vi "TEST.vi"() -> ()   [LabVIEW 2013, in "CConfig Object.lvclass"]
doc: "Copyright 2018, Carya Automatisering, Wiebe Walstra."
uses:
  CConfig Object.lvclass
  Delete Query/Delete Query.lvclass
  Data.ctl
  Loop Query/Loop Query.lvclass
  Insert Query/Insert Query.lvclass
  Composite Query/Composite Query.lvclass
  Step In Query/Step In Query.lvclass
  Add Results Query/Add Results Query.lvclass
  Loop Query/Match Query/Match Query.lvclass
panel:
  out "Index 2":i32
  out "Results":string[][](array[string])
  out "error out":errorcluster
  out "String 3":string
  out "String 2":string
  out "Index out":i32
  out "String":string
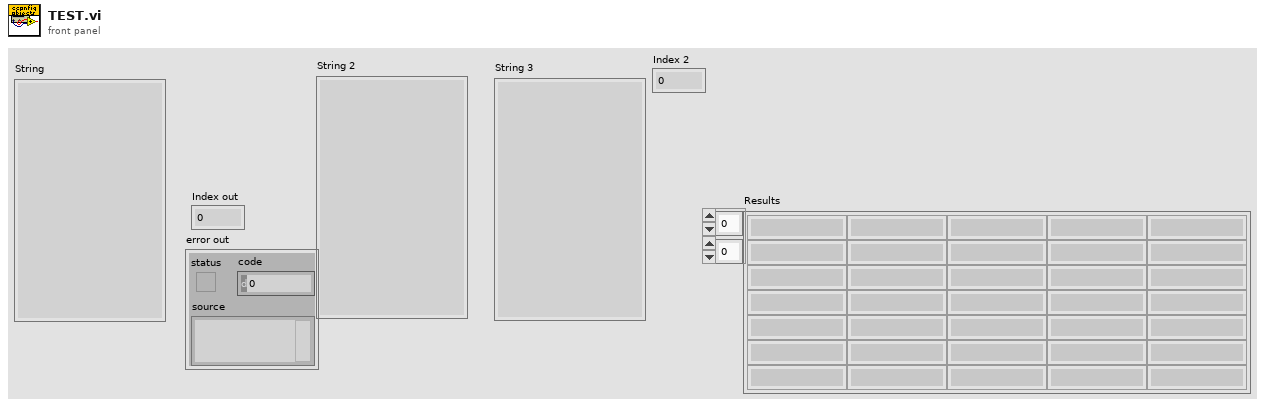
[diagram p1: front panel]
types:
  T1 = typedef "CConfig Object.lvclass/Data.ctl" = enum16{"pre", "name", "middle", "value", "post", "newline", "persistant", "tagged", "type"}
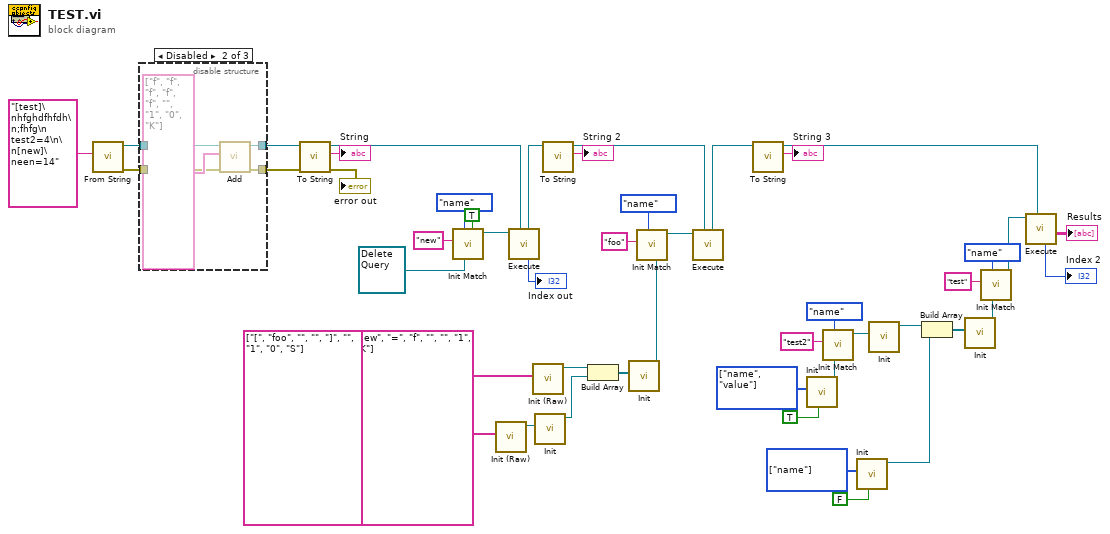
[diagram p0: block diagram]
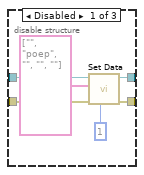
[diagram p2: hidden frame]
diagram:
  w14 = T1[] [enum."name"] items=["pre", "name", "middle", "value", "post", "newline", "persistant", "tagged", "type"] ("Data")
  w26 = T1[] [enum."name", enum."value"] items=["pre", "name", "middle", "value", "post", "newline", "persistant", "tagged", "type"] ("Data")
  n1 = call "From String.vi"("String"="[test]\nhfghdfhfdh\n;fhfg\n test2=4\n\n[new]\neen=14") -> ("error out"=w28:errorcluster, "Section Object out"=w45:refnum<class "CConfig Object.lvclass">)  [unwired: 8 in, 1 out]
  n2 = disable-structure shown="Disabled" {
    disable-tunnel: w45 -> [w53 w58 w60]
    disable-tunnel: [w52 w57 w60] -> w27
    disable-tunnel: [w48 w55 w59] -> w29
    disable-tunnel: w28 -> [w49 w54 w59]
    frame Disabled {
      n3 = call-dynamic "Set Data.vi"("Index in"=1, "error in (no error)"=w49, "Data"=string[] ["", "poep", "", "", ""], "Composite Object in"=w53) -> ("error out"=w48:errorcluster, "Composite Object out"=w52:refnum<class "Config Objects.lvclass">)  [unwired: 6 in]
    }
    frame Disabled {
      n4 = call-dynamic "Add.vi"("error in (no error)"=w54, 10:string[] ["f", "f", "f", "f", "f", "", "1", "0", "K"] ("Data"), "Composite Object in"=w58) -> ("error out"=w55:errorcluster, "Composite Object out"=w57:refnum<class "CConfig Object.lvclass">)  [unwired: 6 in, 1 out]
    }
    frame Enabled {
    }
  }
  n5 = call-dynamic "To String.vi"("error in (no error)"=w29, "Section Object in"=w27) -> ("error out"=→"error out":errorcluster, "String"=→"String":string, "Section Object out"=w1:refnum<class "CConfig Object.lvclass">)  [unwired: 6 in, 1 out]
  n6 = call "Init Match.vi"("Regex [F]"=TRUE, "Found"=refnum<class "Delete Query.lvclass"> refnum ("Delete Query.lvclass"), "Data [name]"=Data."name", "Data"="new") -> ("Find First Query out"=w5:refnum<class "Loop Query.lvclass">)  [unwired: 6 in, 1 out]
  n7 = call "Init (Raw).vi"("Data"=string[] ["", "new", "=", "f", "", "", "1", "0", "K"]) -> ("Find First Query out"=w18:refnum<class "Insert Query.lvclass">)  [unwired: 9 in, 1 out]
  n8 = call-dynamic "Execute.vi"("Composite Object"=w1, "Config Query in"=w5) -> ("Index"=→"Index out":i32, "Composite Object"=w41:refnum<class "CConfig Object.lvclass">)  [unwired: 4 in, 4 out]
  n9 = call "Init (Raw).vi"("Data"=string[] ["[", "foo", "", "", "]", "", "1", "0", "S"]) -> ("Find First Query out"=w32:refnum<class "Insert Query.lvclass">)  [unwired: 9 in, 1 out]
  n10 = call "Init.vi"("Config Query"=w18) -> ("Step In Query out"=w19:refnum<class "Step In Query.lvclass">)  [unwired: 9 in, 1 out]
  n11 = call-dynamic "To String.vi"("Section Object in"=w41) -> ("String"=→"String 2":string, "Section Object out"=w20:refnum<class "CConfig Object.lvclass">)  [unwired: 7 in, 2 out]
  n12 = Build Array(w32, w19) -> (w33:refnum<class "CConfig Query.lvclass">[])
  n13 = call "Init.vi"("Queries"=w33) -> ("Step In Query out"=w34:refnum<class "CConfig Query.lvclass">)  [unwired: 9 in, 1 out]
  n14 = call "Init Match.vi"("Not found"=w34, "Data [name]"=Data."name", "Data"="foo") -> ("Find First Query out"=w4:refnum<class "Loop Query.lvclass">)  [unwired: 7 in, 1 out]
  n15 = call-dynamic "Execute.vi"("Composite Object"=w20, "Config Query in"=w4) -> ("Composite Object"=w36:refnum<class "CConfig Object.lvclass">)  [unwired: 4 in, 5 out]
  n16 = call-dynamic "To String.vi"("Section Object in"=w36) -> ("String"=→"String 3":string, "Section Object out"=w6:refnum<class "CConfig Object.lvclass">)  [unwired: 7 in, 2 out]
  n17 = call "Init.vi"("Concatenate\\Build [T, Concatenate]"=TRUE ("Concatenate\\Build [T, Concatenate]"), "Data [name]"=w26) -> ("Find First Query out"=w13:refnum<class "Add Results Query.lvclass">)  [unwired: 8 in, 1 out]
  n18 = call "Init Match.vi"("Found"=w13, "Data [name]"=Data."name", "Data"="test2") -> ("Find First Query out"=w3:refnum<class "Loop Query.lvclass">)  [unwired: 7 in, 1 out]
  n19 = call "Init.vi"("Concatenate\\Build [T, Concatenate]"=FALSE ("Concatenate\\Build [T, Concatenate]"), "Data [name]"=w14) -> ("Find First Query out"=w9:refnum<class "Add Results Query.lvclass">)  [unwired: 8 in, 1 out]
  n20 = call "Init.vi"("Config Query"=w3) -> ("Step In Query out"=w11:refnum<class "Step In Query.lvclass">)  [unwired: 9 in, 1 out]
  n21 = Build Array(w11, w9) -> (w10:refnum<class "CConfig Query.lvclass">[])
  n22 = call "Init.vi"("Queries"=w10) -> ("Step In Query out"=w12:refnum<class "CConfig Query.lvclass">)  [unwired: 9 in, 1 out]
  n23 = call "Init Match.vi"("Found"=w12, "Data [name]"=Data."name", "Data"="test") -> ("Find First Query out"=w2:refnum<class "Loop Query.lvclass">)  [unwired: 7 in, 1 out]
  n24 = call-dynamic "Execute.vi"("Composite Object"=w6, "Config Query in"=w2) -> ("Results"=→"Results":string[][], "Index"=→"Index 2":i32)  [unwired: 4 in, 4 out]
